vi "Ke2000 DMM Reading.vi"(8 "error in":errorcluster, 11 "VISA In":refnum<visa-resource-name>) -> (0 "error out":errorcluster, 1 "Meas in micro":string, 2 "Read in Micro":dbl, 3 "VISA Out":refnum<visa-resource-name>)   [LabVIEW 2012]
panel:
  out "Units":string
  out "Channel":i32
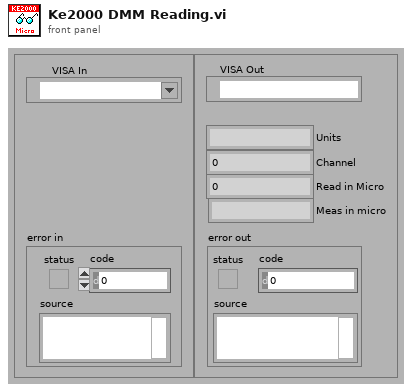
[diagram p1: front panel]
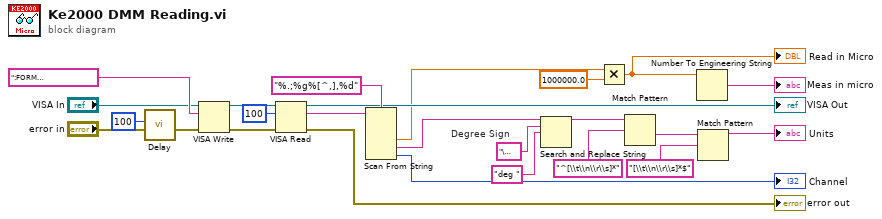
[diagram p0: block diagram]
diagram:
  w12 = "\u0013"  # Degree Sign
  n1 = call "Delay.vi"("error in (no error)"="error in", "milliseconds to wait"=u32 100) -> ("error out"=w7:errorcluster)  [unwired: 9 in]
  n2 = VISA Write(VISA resource name="VISA In", write buffer=":FORM ASC;:FORM:ELEM READ,UNIT,CHAN;:SENS:DATA?", error in (no error)=w7) -> (VISA resource name out=w24:refnum<visa-resource-name>, error out=w23:errorcluster)  [unwired: 1 out]
  n3 = VISA Read(VISA resource name=w24, byte count=u32 100, error in (no error)=w23) -> (VISA resource name out=→"VISA Out":refnum<visa-resource-name>, read buffer=w10:string, error out=→"error out":errorcluster)  [unwired: 1 out]
  n4 = Scan From String(format string="%.;%g%[^,],%d", input string=w10) -> (output 1=w2:dbl, output 2=w13:string, output 3=→"Channel":i32)  [unwired: 5 in, 3 out]
  n5 = Search and Replace String(input string=w13, search string=w12, replace string="deg " ("replace string (\"\")")) -> (result string=w19:string)  [unwired: 5 in, 3 out]
  n6 = Multiply(x=w2, y=1000000.0) -> (x*y=w1:dbl)
  "Read in Micro" <- w1
  n7 = Match Pattern(string=w19, regular expression="^[\\t\\n\\r\\s]*") -> (after substring=w16:string)  [unwired: 1 in, 3 out]
  n8 = Number To Engineering String(4:w1) -> (0:→"Meas in micro":string)  [unwired: 3 in]
  n9 = Match Pattern(string=w16, regular expression="[\\t\\n\\r\\s]*$") -> (before substring=→"Units":string)  [unwired: 1 in, 3 out]
